vi "Init.vi"(10 "Depth":i32=3) -> (3 "Picture out":refnum<class "Picture.lvclass">)   [LabVIEW 2018]
uses:
  Picture.lvclass
  <vilib>/picture/picture.llb/imagedata.ctl
  Coords.ctl
  Picture.lvclass/Picture.ctl
  <vilib>/picture/picture.llb/Draw True-Color Pixmap.vi
panel:
  in  "index (page)":i32
  out "new picture":picture
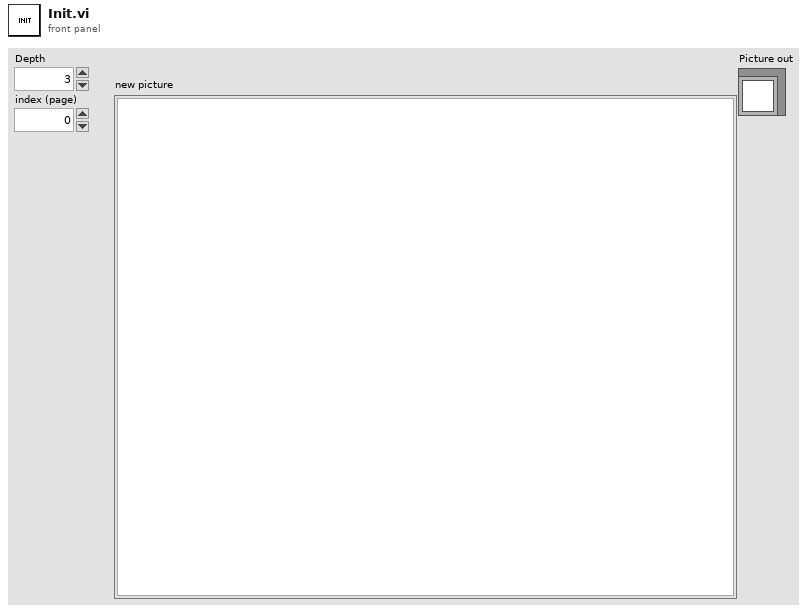
[diagram p1: front panel]
types:
  T1 = typedef "Coords.ctl" = cluster{"Page":i32, "Row":i32, "Column":i32}
  T2 = typedef "imagedata.ctl" = cluster{"image type":i32, "image depth":i32, "image":u8[], "mask":u8[], "colors":u32[], "Rectangle":cluster{"left":i16, "top":i16, "right":i16, "bottom":i16}}
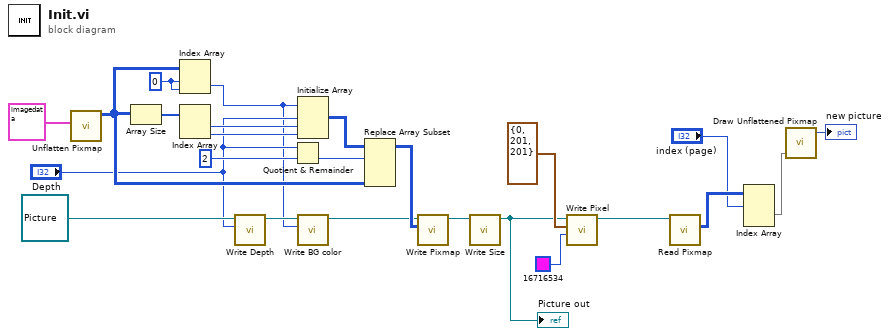
[diagram p0: block diagram]
diagram:
  w22 = 0 ("index (row)")
  n1 = call <vilib>:"Unflatten Pixmap.vi"("image data"=T2 {"image type"=0, "image depth"=24, "image"=array[740862 elements], "mask"=[], "colors"=[], "Rectangle"={"left"=0, "top"=0, "right"=521, "bottom"=474}}) -> ("24-bit pixmap"=w14:u32[][])  [unwired: 4 in, 6 out]
  n2 = Array Size(array=w14) -> (size(s)=w21:i32[])
  n3 = Index Array(array=w14, index (row)=w22, index (col)=w22) -> (element=w6:u32)
  n4 = Index Array(array=w21) -> (element #1=w20:i32, element #2=w19:i32)  [unwired: 2 in]
  n5 = call "Write Depth.vi"("Depth"="Depth", "Picture in"=refnum<class "Picture.lvclass"> refnum ("Picture.lvclass")) -> ("Picture out"=w8:refnum<class "Picture.lvclass">)  [unwired: 8 in, 1 out]
  n6 = Quotient & Remainder(x="Depth", y=2) -> (floor(x/y)=w15:i32)  [unwired: 1 out]
  n7 = Initialize Array(w6, "Depth", w20, w19) -> (w16:u32[][][])
  n8 = call "Write BG color.vi"("BG color"=w6, "Picture in"=w8) -> ("Picture out"=w7:refnum<class "Picture.lvclass">)  [unwired: 8 in, 1 out]
  n9 = Replace Array Subset(array=w16, new element=w14, index (dim 0)=w15) -> (w12:u32[][][])  [unwired: 2 in]
  n10 = call "Write Pixmap.vi"("3D Pixmap"=w12, "Picture in"=w7) -> ("Picture out"=w2:refnum<class "Picture.lvclass">)  [unwired: 8 in, 1 out]
  n11 = call "Write Size.vi"("Picture in"=w2) -> ("Picture out"=w1:refnum<class "Picture.lvclass">)  [unwired: 9 in, 1 out]
  "Picture out" <- w1
  n12 = call "Write Pixel.vi"("Color"=u32 16716534, "indices"=T1 {"Page"=0, "Row"=201, "Column"=201}, "Picture in"=w1) -> ("Picture out"=w4:refnum<class "Picture.lvclass">)  [unwired: 7 in, 1 out]
  n13 = call "Read Pixmap.vi"("Picture in"=w4) -> ("3D Pixmap"=w11:u32[][][])  [unwired: 8 in, 2 out]
  n14 = Index Array(array=w11, index (dim 0)="index (page)") -> (element=w9:u32[][])  [unwired: 2 in]
  n15 = call-poly <vilib>:"Draw Unflattened Pixmap.vi"("data (RGB format)"=w9) -> ("new picture"=→"new picture":picture)  [unwired: 8 in]
